vi "Shut Down Device.vi"(8 "error in (no error)":errorcluster, 11 "Synchronization Device in":refnum<class "Sync Device.lvclass">) -> (0 "error out":errorcluster, 3 "Synchronization Device out":refnum<class "Sync Device.lvclass">)   [LabVIEW 2023, in "Sync Device.lvlib" / "Sync Device.lvclass"]
uses:
  Sync Device.lvclass
  Sync Device.lvclass/Sync Device.ctl
  <vilib>/DAQmx/miscellaneous.llb/DAQmx Fill In Error Info.vi
  Device/Device.lvclass
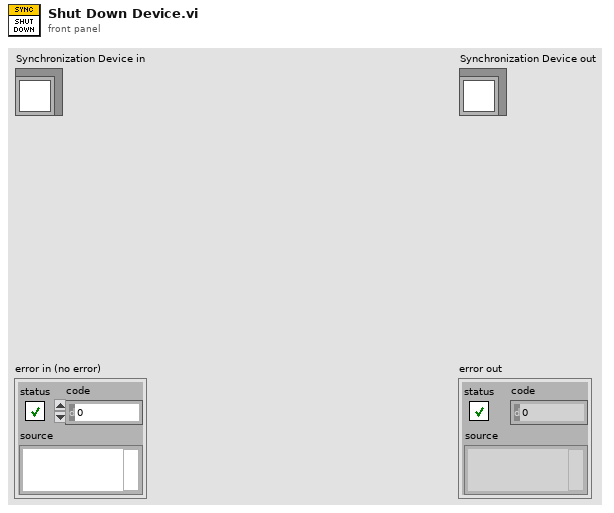
[diagram p1: front panel]
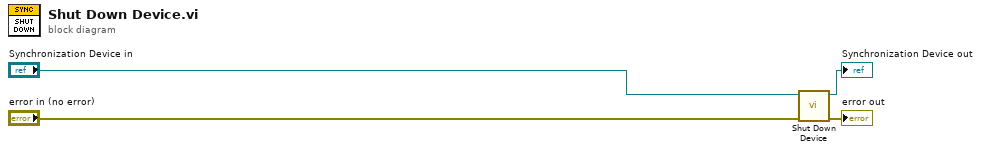
[diagram p0: block diagram]
diagram:
  n1 = call-parent "Shut Down Device.vi"("error in (no error)"="error in (no error)", "Device in"="Synchronization Device in") -> ("error out"=→"error out":errorcluster, "Device out"=→"Synchronization Device out":refnum<class "Sync Device.lvclass">)  [unwired: 8 in]
